vi "CheckSelectionStability.vi"() -> ()   [LabVIEW 2016]
uses:
  MFCdescription.ctl
  MFCcapability.ctl
panel:
  in  "MFCcapabilities":T1[](array[typedef]) {"mDot" format="%_4g"; "Setpoint" format="%.2g"; "MFCcapability"."MaxMdot" format="%_4g"; "MFCcapability"."MinMdot" format="%_4g"}
  in  "Max":dbl=350.0 format="%#_13g"
  in  "Increment":dbl=1.0
  out "XY Graph":cluster{dbl[], dbl[]}[](graph)
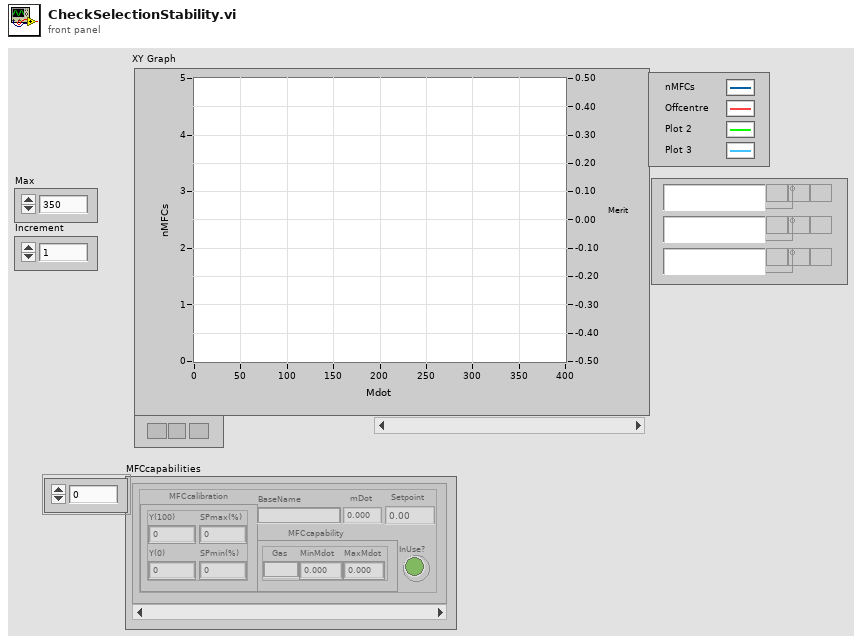
[diagram p1: front panel]
types:
  T1 = typedef "MFCdescription.ctl" = cluster{"BaseName":string, "MFCcalibration":cluster{"Y(100)":dbl, "Y(0)":dbl, "SPmin(%)":dbl, "SPmax(%)":dbl}, "MFCcapability":T2, "InUse?":bool, "Setpoint":dbl, "mDot":dbl}
  T2 = typedef "MFCcapability.ctl" = cluster{"Gas":string, "MinMdot":dbl, "MaxMdot":dbl}
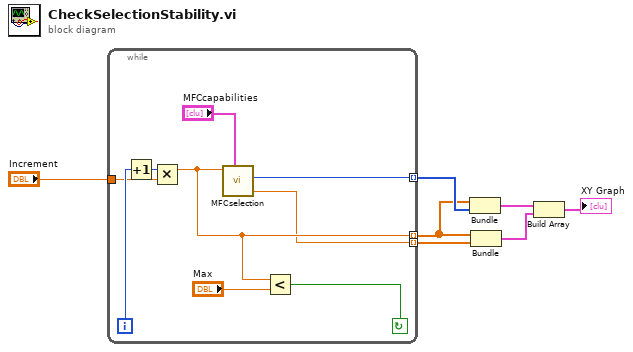
[diagram p0: block diagram]
diagram:
  n1 = while {
    tunnel: [w16] -> w7 mode=indexing
    tunnel: [w13] -> w4 mode=indexing
    tunnel: "Increment" -> [w14]
    tunnel: [w10] -> w3 mode=indexing
    i -> [w15]
    stop <- w11 continue-if-true
    n2 = Increment(x=w15) -> (x+1=w9:i32)
    n3 = Multiply(x=w9, y=w14) -> (x*y=w13:dbl)
    n4 = call "MFCselection.vi"("MFCsIn"="MFCcapabilities", "Mdot"=w13) -> ("OffCentre"=w10:dbl, "nMFCs"=w16:i32)  [unwired: 4 in, 2 out]
    n5 = Less?(x=w13, y="Max") -> (x < y?=w11:bool)
  }
  n6 = Bundle(w4, w7) -> (w6:cluster{dbl[], i32[]})  [unwired: 1 in]
  n7 = Bundle(w4, w3) -> (w1:cluster{dbl[], dbl[]})  [unwired: 1 in]
  n8 = Build Array(w6, w1) -> (→"XY Graph":cluster{dbl[], dbl[]}[])
